vi "Finish.vi"   [LabVIEW 2019]
doc: "This VI is called just before exiting. It is expected to close I/O refnum, save collected data, etc."
uses:
  <vilib>/Rock Robotics/WPI/Utilities/WPI_GetSetVariantRefNum.vi
types:
  T1 = typedef "WPI_JoystickDevRef.ctl" = cluster{"Device":T2}
  T2 = typedef "WPI_JoystickDeviceEnum.ctl" = enum16{"USB 0", "USB 1", "USB 2", "USB 3", "USB 4", "USB 5"}
  T3 = typedef "WPI_RobotDriveDevRef.ctl" = cluster{"DevStatus":errorcluster, "Motors[]":T4[], "Square Inputs":bool, "Max Output":dbl}
  T4 = typedef "WPI_MotorControlDeviceRef.ctl" = cluster{"DeviceStatus":errorcluster, "Type":T5, "PWM":cluster{"PWM Channel":T6, "DeadBand":T7}, "CAN":cluster{"Device Number":u8, "SetOutput VI Ref":variant, "GetOutput VI Ref":variant, "Enable VI Ref":variant, "Disable VI Ref":variant, "Data":variant}, "Invert":bool, "DIO PWM":cluster{"PWM \"Enable\" Channel":T6, "DIOChannel":T8, "PWM Rate":dbl}}
  T5 = typedef "WPI_MotorControlType.ctl" = enum16{"PWM", "CAN", "DIO PWM"}
  T6 = typedef "FPGA_DIOPWMChannel.ctl" = enum8{"PWM 0", "PWM 1", "PWM 2", "PWM 3", "PWM 4", "PWM 5", "PWM 6", "PWM 7", "PWM 8", "PWM 9", "PWM MXP 0", "PWM MXP 1", "PWM MXP 2", "PWM MXP 3", "PWM MXP 4", "PWM MXP 5", "PWM MXP 6", "PWM MXP 7", "PWM MXP 8", "PWM MXP 9", "Invalid"}
  T7 = typedef "WPI_PWMDeadband.ctl" = cluster{"Name":string, "maxPositivePwm":i32, "minPositivePwm":i32, "centerPwm":i32, "maxNegativePwm":i32, "minNegativePwm":i32, "angularRange":u16}
  T8 = typedef "FPGA_DIOChannel.ctl" = enum8{"DIO 0", "DIO 1", "DIO 2", "DIO 3", "DIO 4", "DIO 5", "DIO 6", "DIO 7", "DIO 8", "DIO 9", "DIO MXP 0", "DIO MXP 1", "DIO MXP 2", "DIO MXP 3", "DIO MXP 4", "DIO MXP 5", "DIO MXP 6", "DIO MXP 7", "DIO MXP 8", "DIO MXP 9", "DIO MXP 10", "DIO MXP 11", "DIO MXP 12", "DIO MXP 13", "DIO MXP 14", "DIO MXP 15", "SPI Port CS1", "SPI Port CS2", "SPI Port CS3", "SPI Port MISO", "SPI Port MOSI", "Invalid"}
  T9 = typedef "WPI_GyroDevRef.ctl" = cluster{"DevStatus":errorcluster, "Analog Channel":T10, "Gain (VoltsPerDegree/Second)":dbl, "Gyro Type":enum16{"Analog", "XRS450"}, "Handle":i32, "SPI Bus":T11, "Device Found":bool, "Sample Rate":dbl, "Calibrate On Open":bool, "Offset":dbl}
  T10 = typedef "FPGA_AIChannel.ctl" = enum8{"AI 0", "AI 1", "AI 2", "AI 3", "AI MXP 0", "AI MXP 1", "AI MXP 2", "AI MXP 3", "Invalid"}
  T11 = typedef "spi_bus.ctl" = enum16{"SPI On-Board, CS0", "SPI On-Board, CS1", "SPI On-Board, CS2", "SPI On-Board, CS3", "SPI MXP", "Invalid"}
  T12 = typedef "Color Sensor V3 DevRef.ctl" = cluster{"I2CDevRef":T13}
  T13 = typedef "WPI_I2CDevRef.ctl" = cluster{"DevStatus":errorcluster, "Device Address":u8, "Handle":i32, "I2C Bus":T14}
  T14 = typedef "i2c_bus.ctl" = enum16{"I2C On-Board", "I2C MXP", "Invalid"}
  T15 = typedef "WPI_SwitchDevRef.ctl" = cluster{"DevStatus":errorcluster, "DIO Channel":T8, "CntIndex":T16, "Normally Closed":bool}
  T16 = typedef "FPGA_CounterCtrSystemIndex.ctl" = enum8{"Ctr 0", "Ctr 1", "Ctr 2", "Ctr 3", "Ctr 4", "Ctr 5", "Ctr 6", "Ctr 7", "Invalid"}
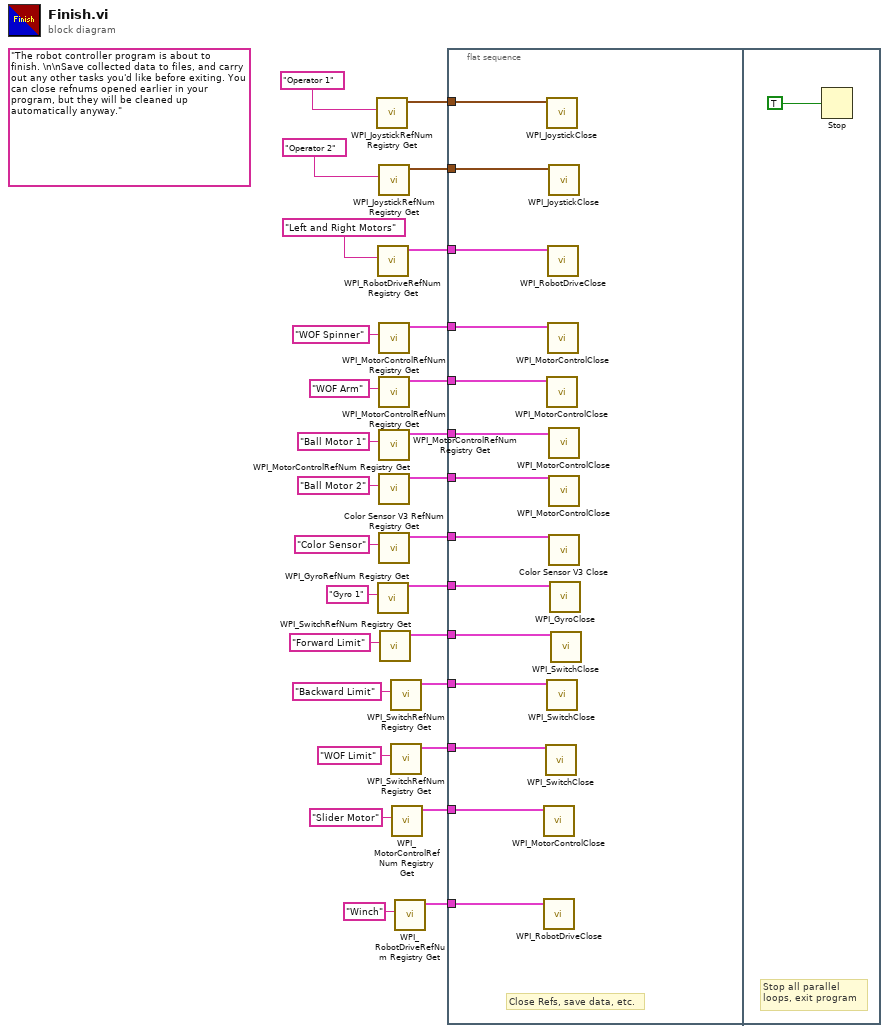
[diagram p0: block diagram]
diagram:
  (unwired) "The robot controller program is about to finish. \n\nSave collected data to files, and carry out any other tasks you'd like before exiting. You can close refnums opened earlier in your program, but they will be cleaned up automatically anyway."
  n1 = call <vilib>:"WPI_JoystickRefNum Registry Get.vi"("refnum name"="Operator 1") -> ("JoystickDevRef"=w25:T1)  [unwired: 1 in, 9 out]
  n2 = call <vilib>:"WPI_RobotDriveRefNum Registry Get.vi"("refnum name"="Left and Right Motors") -> ("RobotDriveDevRef"=w26:T3)  [unwired: 1 in, 9 out]
  n3 = call <vilib>:"WPI_GyroRefNum Registry Get.vi"("refnum name"="Gyro 1") -> ("GyroDevRef"=w15:T9)  [unwired: 9 in, 1 out]
  n4 = call <vilib>:"WPI_JoystickRefNum Registry Get.vi"("refnum name"="Operator 2") -> ("JoystickDevRef"=w4:T1)  [unwired: 1 in, 9 out]
  n5 = call <vilib>:"WPI_MotorControlRefNum Registry Get.vi"("refnum name"="WOF Spinner") -> ("MotorControlDevRef"=w20:T4)  [unwired: 9 in, 1 out]
  n6 = call <vilib>:"WPI_MotorControlRefNum Registry Get.vi"("refnum name"="WOF Arm") -> ("MotorControlDevRef"=w6:T4)  [unwired: 9 in, 1 out]
  n7 = call <vilib>:"WPI_MotorControlRefNum Registry Get.vi"("refnum name"="Ball Motor 1") -> ("MotorControlDevRef"=w24:T4)  [unwired: 9 in, 1 out]
  n8 = call <vilib>:"WPI_MotorControlRefNum Registry Get.vi"("refnum name"="Ball Motor 2") -> ("MotorControlDevRef"=w22:T4)  [unwired: 9 in, 1 out]
  n9 = call <vilib>:"Color Sensor V3 RefNum Registry Get.vi"("refnum name"="Color Sensor") -> ("ColorSensorDevRef"=w18:T12)  [unwired: 9 in, 1 out]
  n10 = call <vilib>:"WPI_SwitchRefNum Registry Get.vi"("refnum name"="Forward Limit") -> ("SwitchDevRef"=w14:T15)  [unwired: 9 in, 1 out]
  n11 = call <vilib>:"WPI_SwitchRefNum Registry Get.vi"("refnum name"="Backward Limit") -> ("SwitchDevRef"=w11:T15)  [unwired: 9 in, 1 out]
  n12 = call <vilib>:"WPI_SwitchRefNum Registry Get.vi"("refnum name"="WOF Limit") -> ("SwitchDevRef"=w10:T15)  [unwired: 9 in, 1 out]
  n13 = call <vilib>:"WPI_MotorControlRefNum Registry Get.vi"("refnum name"="Slider Motor") -> ("MotorControlDevRef"=w8:T4)  [unwired: 9 in, 1 out]
  n14 = call <vilib>:"WPI_RobotDriveRefNum Registry Get.vi"("refnum name"="Winch") -> ("RobotDriveDevRef"=w2:T3)  [unwired: 9 in, 1 out]
  n15 = flat-sequence {
    tunnel: w26 -> [w42]
    tunnel: w25 -> [w41]
    tunnel: w24 -> [w40]
    tunnel: w22 -> [w39]
    tunnel: w20 -> [w38]
    tunnel: w18 -> [w37]
    tunnel: w15 -> [w36]
    tunnel: w14 -> [w35]
    tunnel: w11 -> [w34]
    tunnel: w10 -> [w33]
    tunnel: w8 -> [w32]
    tunnel: w6 -> [w31]
    tunnel: w4 -> [w30]
    tunnel: w2 -> [w29]
    frame #0 {
      # "Close Refs, save data, etc."
      n16 = call <vilib>:"WPI_MotorControlClose.vi"("MotorControlDevRef"=w32) -> ()  [unwired: 10 in, 1 out]
      n17 = call <vilib>:"WPI_RobotDriveClose.vi"("RobotDriveDevRef"=w29) -> ()  [unwired: 10 in, 1 out]
      n18 = call <vilib>:"WPI_SwitchClose.vi"("SwitchDevRef"=w33) -> ()  [unwired: 10 in, 1 out]
      n19 = call <vilib>:"WPI_JoystickClose.vi"("JoystickDevRef"=w41) -> ()  [unwired: 11 out]
      n20 = call <vilib>:"WPI_MotorControlClose.vi"("MotorControlDevRef"=w31) -> ()  [unwired: 10 in, 1 out]
      n21 = call <vilib>:"WPI_SwitchClose.vi"("SwitchDevRef"=w34) -> ()  [unwired: 10 in, 1 out]
      n22 = call <vilib>:"WPI_RobotDriveClose.vi"("RobotDriveDevRef"=w42) -> ()  [unwired: 1 in, 10 out]
      n23 = call <vilib>:"WPI_MotorControlClose.vi"("MotorControlDevRef"=w38) -> ()  [unwired: 10 in, 1 out]
      n24 = call <vilib>:"WPI_JoystickClose.vi"("JoystickDevRef"=w30) -> ()  [unwired: 11 out]
      n25 = call <vilib>:"WPI_MotorControlClose.vi"("MotorControlDevRef"=w40) -> ()  [unwired: 10 in, 1 out]
      n26 = call <vilib>:"WPI_MotorControlClose.vi"("MotorControlDevRef"=w39) -> ()  [unwired: 10 in, 1 out]
      n27 = call <vilib>:"Color Sensor V3 Close.vi"("ColorSensorDevRef in"=w37) -> ()  [unwired: 10 in, 1 out]
      n28 = call <vilib>:"WPI_GyroClose.vi"("GyroDevRef"=w36) -> ()  [unwired: 10 in, 1 out]
      n29 = call <vilib>:"WPI_SwitchClose.vi"("SwitchDevRef"=w35) -> ()  [unwired: 10 in, 1 out]
    }
    frame #1 {
      # "Stop all parallel\nloops, exit program"
      n30 = Stop(stop? (T)=TRUE ("Quit")) -> ()
    }
  }
